vi "fake tool return error.vi"(9 "source":string, 10 "code":i32, 11 "status":bool) -> (0 "error out":errorcluster)   [LabVIEW 2020, in "MCP Server tests.lvlib"]
doc: "this is a test tool that returns an error cluster."
uses:
  MCP Server tests.lvlib
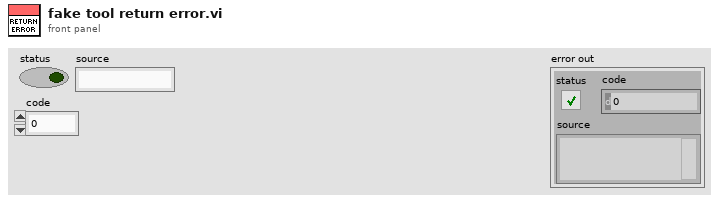
[diagram p1: front panel]
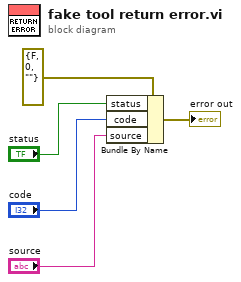
[diagram p0: block diagram]
diagram:
  n1 = Bundle By Name(cluster=errorcluster {"status"=FALSE, "code"=0, "source"=""} ("error constant"), "status"="status", "code"="code", "source"="source") -> (→"error out":errorcluster)
